vi "DAC-selector.vi"(8 "data-in":fxp<+/-,20,5>, 11 "DAC-select":i16(ring) items=["Mod2/AO0", "Mod2/AO1", "Mod2/AO2", "Mod2/AO3", ""]) -> ()   [LabVIEW 2017]
uses:
  <vilib>/rvi/eio/common/nirviEmuTemplateMethod_errors.vi
  <vilib>/eio/EIONode/EIONode.xnode
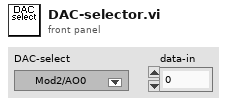
[diagram p1: front panel]
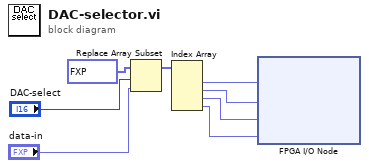
[diagram p0: block diagram]
diagram:
  n1 = Replace Array Subset(array=fxp<+/-,20,5>[] [0.0, 0.0, 0.0, 0.0], new element="data-in", index="DAC-select") -> (w4:fxp<+/-,20,5>[])
  n2 = Index Array(array=w4) -> (element #1=w8:fxp<+/-,20,5>, element #2=w7:fxp<+/-,20,5>, element #3=w6:fxp<+/-,20,5>, element #4=w5:fxp<+/-,20,5>)  [unwired: 4 in]
  n3 = xnode "FPGA I/O Node"("Mod1/AO0"=w8, "Mod1/AO1"=w7, "Mod1/AO2"=w6, "Mod1/AO3"=w5) -> ()  [unwired: 4 in, 4 out]
